vi "MOCK_FP_Write_Double_Array.vi"(8 "error in":errorcluster, 9 "on change (false)":bool, 10 "values":dbl[](array[numeric]) format="%.2f", 11 "FieldPoint IO Point In":refnum<k21>) -> (0 "error out":errorcluster, 2 "timestamp":dbl format="%.2f", 3 "FieldPoint IO Point Out":refnum<k21>)   [LabVIEW 2017]
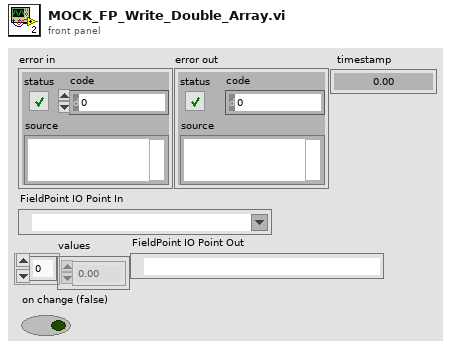
[diagram p1: front panel]
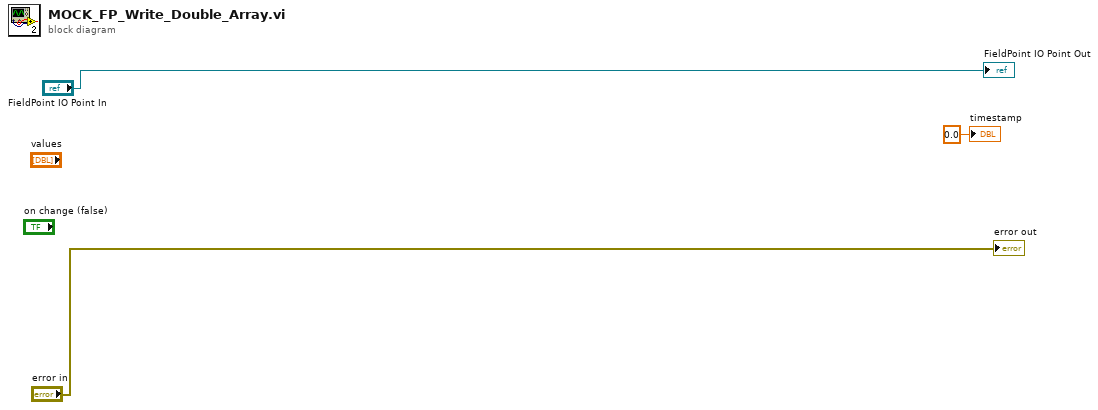
[diagram p0: block diagram]
diagram:
  "error out" <- "error in"
  "timestamp" <- 0.0 ("timestamp")
  "FieldPoint IO Point Out" <- "FieldPoint IO Point In"
